vi "I2C Read Write.vi"(0 "handle":u32 format="%08x", 5 "deviceAddress":u32 format="%x", 7 "String":string="To", 11 "error in (no error)":errorcluster) -> (4 "handle out":u32 format="%08x", 6 "sizeTransferred":u32, 15 "error out":errorcluster)   [LabVIEW 2024, in "libMPSSE-I2C.lvlib"]
doc: "FTDI_API FT_STATUS SPI_ReadWrite(FT_HANDLE handle, uint8 *inBuffer,\n uint8 *outBuffer, uint32 sizeToTransfer, uint32 *sizeTransferred,\n uint32 transferOptions);"
uses:
  libMPSSE-I2C.lvlib
  libmpsse.dll
panel:
  in  "*buffer 3":u8[](array[numeric]) format="%x"
  in  "sizeToTransfer 3":u32
  in  "*buffer 2":u8[](array[numeric]) format="%x"
  out "return type":u32
  out "sizeToTransfer":u32
  out "error out 2":errorcluster
  in  "error in (no error) 2":errorcluster
  out "sizeTransferred 2":u32
  in  "options":u32=6 format="%x"
  # "/* transferOptions-Bit0: If this bit is 0 then it means that the transfer size provided is in bytes */\n#define\tSPI_TRANSFER_OPTIONS_SIZE_IN_BYTES\t\t\t0x00000000\n/* transferOptions-Bit0: If this bit is 1 then it means that the transfer size provided is in bytes */\n#define\tSPI_TRANSFER_OPTIONS_SIZE_IN_BITS\t\t\t0x00000001\n/* transferOptions-Bit1: if BIT1 is 1 then CHIP_SELECT line will be enabled at start of transfer */\n#define\tSPI_TRANSFER_OPTIONS_CHIPSELECT_ENABLE\t\t0x00000002\n/* transferOptions-Bit2: if BIT2 is 1 then CHIP_SELECT line will be disabled at end of transfer */\n#define SPI_TRANSFER_OPTIONS_CHIPSELECT_DISABLE\t\t0x00000004"
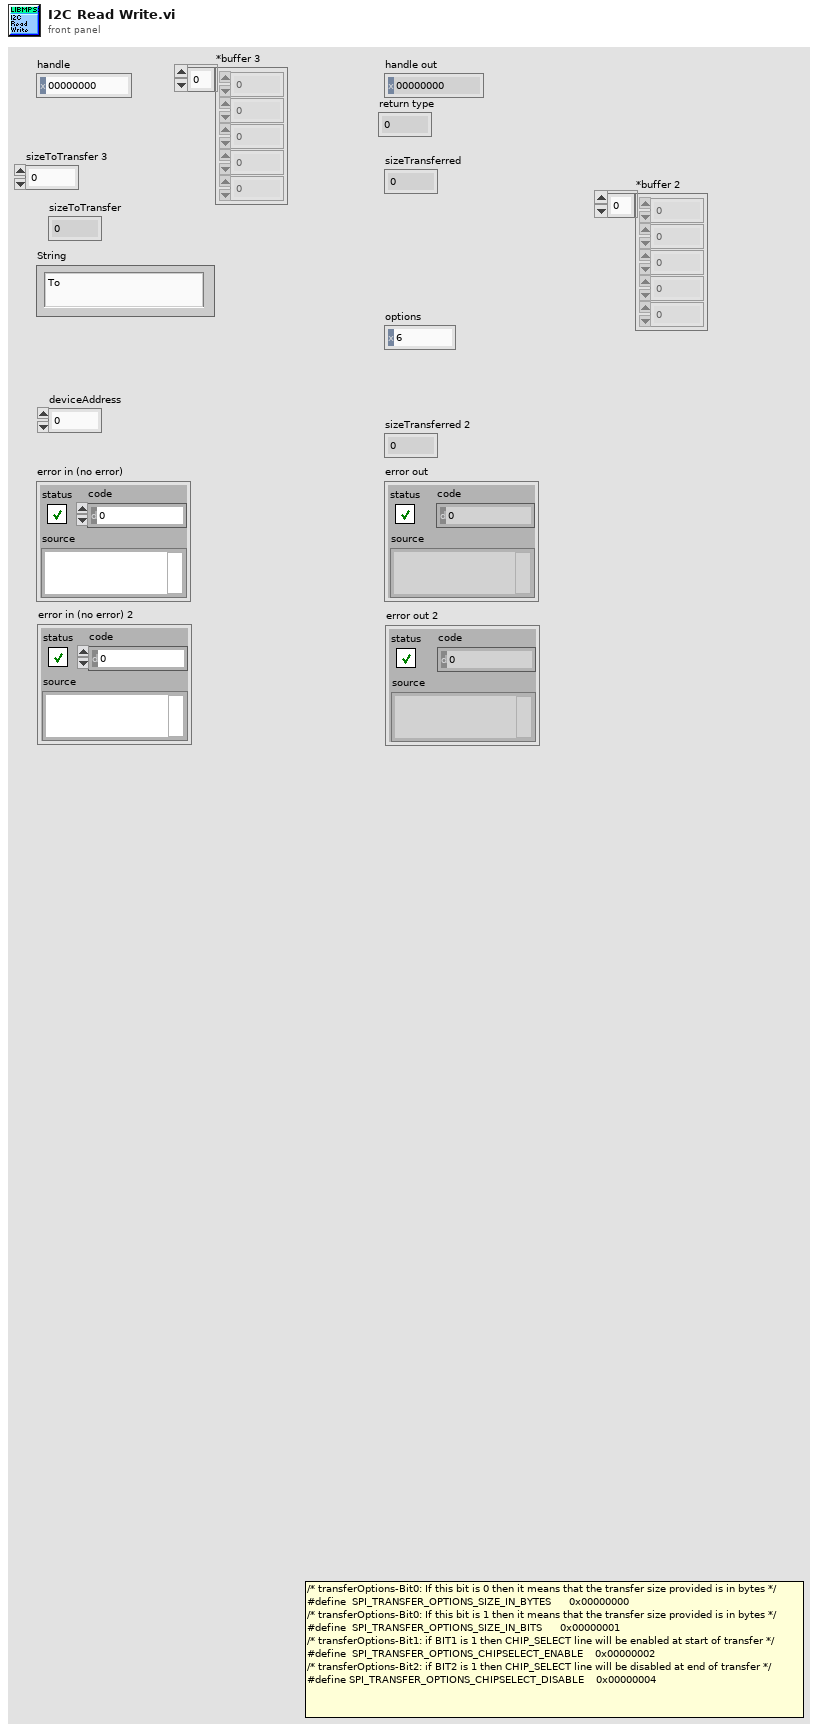
[diagram p1: front panel]
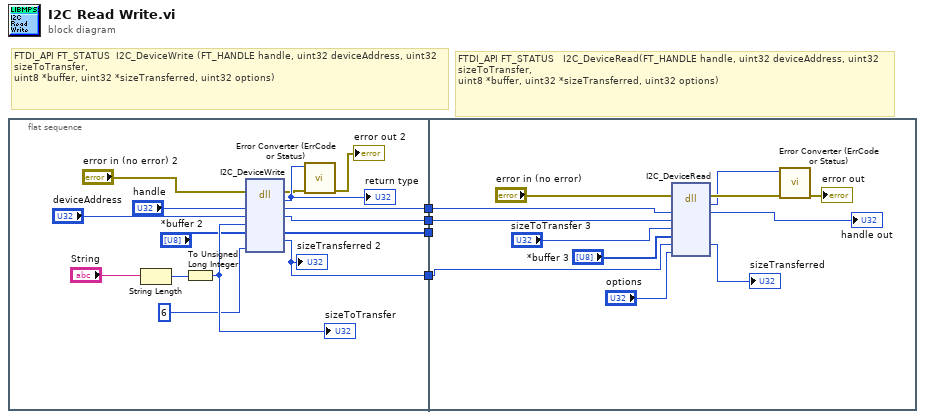
[diagram p0: block diagram]
diagram:
  # "FTDI_API FT_STATUS   I2C_DeviceRead(FT_HANDLE handle, uint32 deviceAddress, uint32 sizeToTransfer, \nuint8 *buffer, uint32 *sizeTransferred, uint32 options)"
  # "FTDI_API FT_STATUS  I2C_DeviceWrite (FT_HANDLE handle, uint32 deviceAddress, uint32 sizeToTransfer, \nuint8 *buffer, uint32 *sizeTransferred, uint32 options)"
  n1 = flat-sequence {
    tunnel: [w13] -> w4
    tunnel: [w10] -> w3
    tunnel: [w9] -> w2
    tunnel: [w7] -> w1
    tunnel: w4 -> [_]
    tunnel: w3 -> [w24]
    tunnel: w2 -> [w23]
    tunnel: w1 -> [w22]
    frame #0 {
      n2 = String Length(string="String") -> (length=w12:i32)
      n3 = To Unsigned Long Integer(number=w12) -> (unsigned 32bit integer=w8:u32)
      "sizeToTransfer" <- w8
      n4 = dll-call lib="C:/Workspace/sm_6576_001_RIB_Sequencer/I2C/libMPSSE.*" fn="I2C_DeviceWrite"(error in="error in (no error) 2", "handle"="handle", "deviceAddress"="deviceAddress", "sizeToTransfer"=w8, "*buffer"="*buffer 2", "options"=u32 6) -> (error out=w16:errorcluster, "return type"=w19:u32, "handle"=w10:u32, "deviceAddress"=w9:u32, "*buffer"=w13:u8[], "*sizeTransferred"=w7:u32)  [unwired: 5 in, 1 out]
      "sizeTransferred 2" <- w7
      "return type" <- w19
      n5 = call "Error Converter (ErrCode or Status).vi"("error in (no error)"=w16, "error code"=w19) -> ("error out"=→"error out 2":errorcluster)  [unwired: 9 in]
    }
    frame #1 {
      n6 = dll-call lib="C:/Workspace/sm_6576_001_RIB_Sequencer/I2C/libMPSSE.*" fn="I2C_DeviceRead"(error in="error in (no error)", "handle"=w24, "deviceAddress"=w23, "sizeToTransfer"="sizeToTransfer 3", "*buffer"="*buffer 3", "*sizeTransferred"=w22, "options"="options") -> (error out=w28:errorcluster, "return type"=w25:u32, "handle"=→"handle out":u32, "*sizeTransferred"=→"sizeTransferred":u32)  [unwired: 6 in, 1 out]
      n7 = call "Error Converter (ErrCode or Status).vi"("error in (no error)"=w28, "error code"=w25) -> ("error out"=→"error out":errorcluster)  [unwired: 9 in]
    }
  }
